vi "Execute.vi"(8 "error in":errorcluster, 10 "Command in":refnum<class "Command.lvclass">, 11 "Instrument In":refnum<class>) -> (0 "error out":errorcluster, 3 "Instrument Out":refnum<class>)   [LabVIEW 2015, in "Command.lvclass"]
uses:
  Command.lvclass
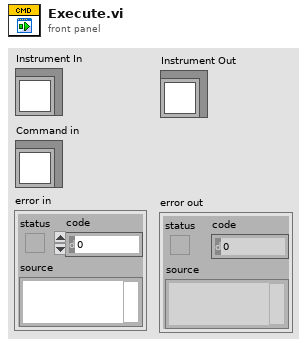
[diagram p1: front panel]
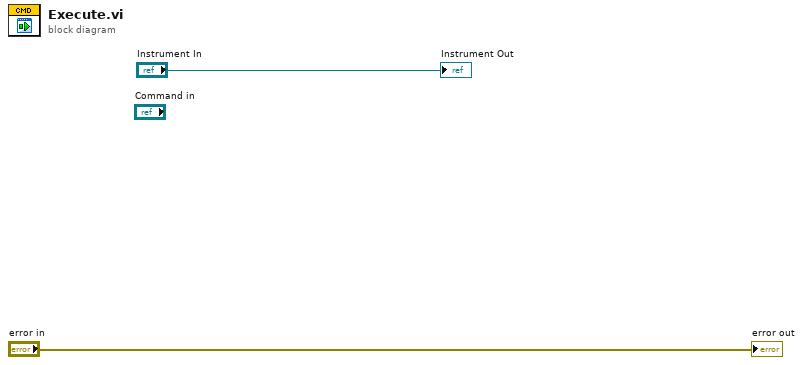
[diagram p0: block diagram]
diagram:
  "error out" <- "error in"
  "Instrument Out" <- "Instrument In"
